vi "Load_from_Project.vi"(8 "error in (no error)":errorcluster, 9 "index":string, 10 "buildObject":T1, 11 "IB_Shortcut in":refnum<class "IB_Shortcut.lvclass">) -> (0 "error out":errorcluster, 1 "index out":string, 2 "buildObject out":T1, 3 "IB_Shortcut out":refnum<class "IB_Shortcut.lvclass">)   [LabVIEW 2020, in "IB_Shortcut.lvclass"]
uses:
  <vilib>/AppBuilder/IB_Classes/Shortcut/IB_Shortcut.lvclass
  <vilib>/AppBuilder/IB_Classes/Shortcut/IB_Shortcut.lvclass/IB_Shortcut.ctl
  <vilib>/AppBuilder/IB_RW_Project/IB_RW_Project_PropBag_Action.ctl
  <resource>/Framework/Providers/API/ItemRef.ctl
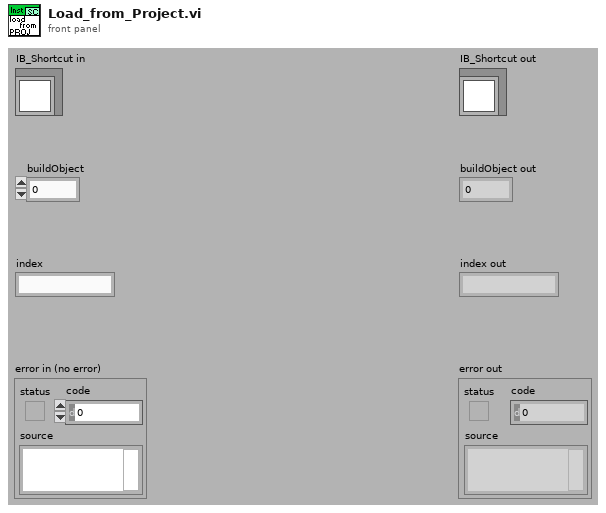
[diagram p1: front panel]
types:
  T1 = typedef "ItemRef.ctl" = u64
  T2 = typedef "IB_RW_Project_PropBag_Action.ctl" = enum16{"read", "write", "clear", "readPrevious", "writePrevious", "clearPrevious"}
  T3 = typedef "IB_RW_Project_Shortcut_Data.ctl" = cluster{"name":string, "destIndex":i32, "subDir":string}
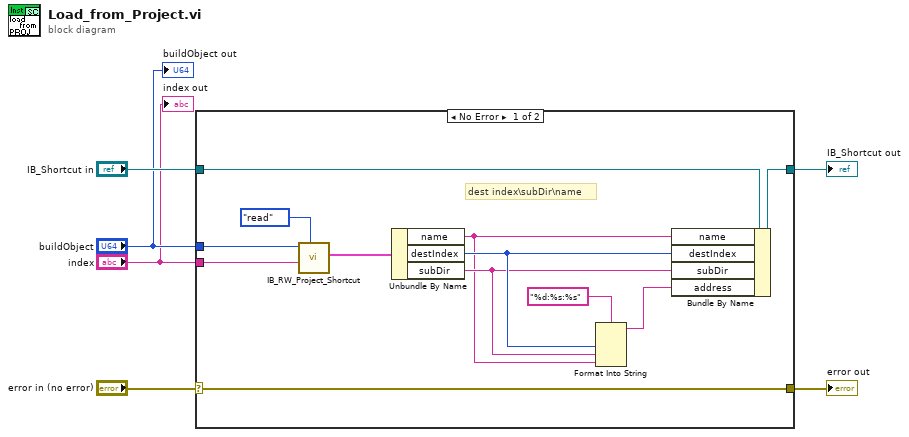
[diagram p0: block diagram]
diagram:
  n1 = case shown="No Error" "error in (no error)" {
    selector: "error in (no error)" -> [w18 w20]
    tunnel: [w18 w20] -> w5
    tunnel: [w12 w19] -> w3
    tunnel: "IB_Shortcut in" -> [w13 w19]
    tunnel: "index" -> [w16 _]
    tunnel: "buildObject" -> [w15 _]
    frame No Error {
      # "dest index\\subDir\\name"
      n2 = call <vilib>:"IB_RW_Project_Shortcut.vi"("action"=IB_RW_Project_PropBag_Action."read", "index in"=w16, "buildObject"=w15) -> ("dataSource out"=w14:T3)  [unwired: 2 in, 6 out]
      n3 = Unbundle By Name(w14) -> ("name"=w8:string, "destIndex"=w10:i32, "subDir"=w9:string)
      n4 = Format Into String(format string="%d:%s:%s", w10, w9, w8) -> (resulting string=w7:string)  [unwired: 2 in, 1 out]
      n5 = Bundle By Name(cluster=w13, "name"=w8, "destIndex"=w10, "subDir"=w9, "address"=w7) -> (w12:refnum<class "IB_Shortcut.lvclass">)
    }
    frame Error {
    }
  }
  "error out" <- w5
  "IB_Shortcut out" <- w3
  "buildObject out" <- "buildObject"
  "index out" <- "index"
